vi "AutoBalance.vi"(8 "error in (no error)":errorcluster) -> (0 "error out":errorcluster)   [LabVIEW 2020]
doc: "Wrapper class for drive straight"
uses:
  <vilib>/Utility/semaphor.llb/Obtain Semaphore Reference.vi
  <vilib>/Rock Robotics/WPI/ThirdParty/JAS_Junk/TrajLib/Timer_Reset.vi
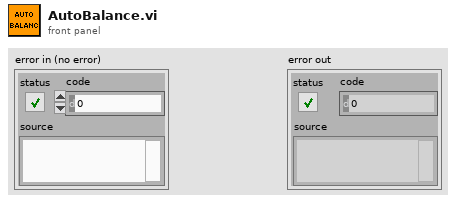
[diagram p1: front panel]
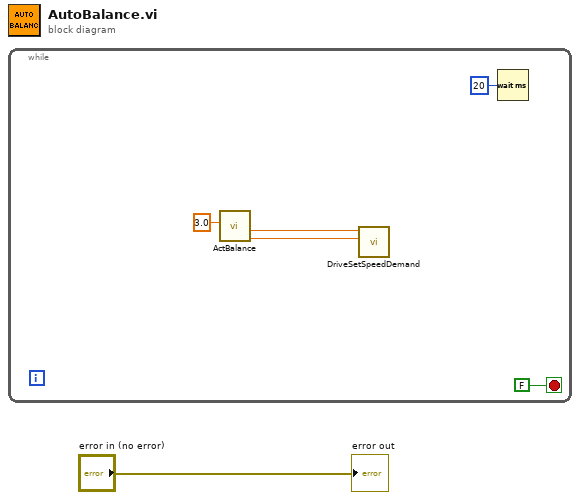
[diagram p0: block diagram]
diagram:
  n1 = while {
    stop <- FALSE stop-if-true
    n2 = call "ActBalance.vi"("MaxSpeed (ft/s)"=3.0) -> ("RightSpeedDemand"=w3:dbl, "LeftSpeedDemand"=w4:dbl)  [unwired: 8 in, 1 out]
    n3 = call "DriveSetSpeedDemand.vi"("RSpeedDemand (ft/s)"=w3, "LSpeedDemand (ft/s)"=w4) -> ()  [unwired: 10 in]
    n4 = Wait (ms)(milliseconds to wait=u32 20) -> ()  [unwired: 1 out]
  }
  "error out" <- "error in (no error)"
